vi "Configure List Save Or Recall.vi"(8 "error in":errorcluster, 9 "File Name":u8=1 min=1 max=10 step=1, 10 "Save Or Recall":u16(ring) items=["Save", "Recall"], 11 "VISA resource name":refnum<visa-resource-name>) -> (0 "error out":errorcluster, 3 "VISA resource name out":refnum<visa-resource-name>)   [LabVIEW 2018, in "IT-M3100.lvlib"]
doc: "This command is set to save or recall list file.\n<b>Save Or Recall</b>\n0:Save:This command saves the present list program into the specified memory.\n1:Recall:This command recalls the list program you saved in the specified memory location.\n<b>File Name</b>\n1-10"
uses:
  IT-M3100.lvlib
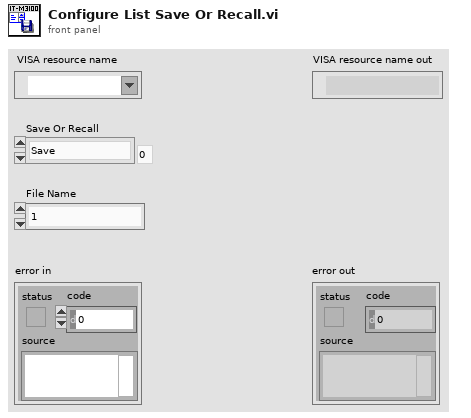
[diagram p1: front panel]
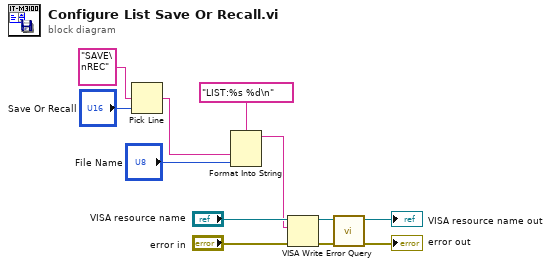
[diagram p0: block diagram]
diagram:
  n1 = Pick Line(multi-line string="SAVE\nREC", line index="Save Or Recall") -> (output string=w1:string)  [unwired: 1 in]
  n2 = Format Into String(format string="LIST:%s %d\n", w1, "File Name") -> (resulting string=w5:string)  [unwired: 2 in, 1 out]
  n3 = VISA Write(VISA resource name="VISA resource name", write buffer=w5, error in (no error)="error in") -> (VISA resource name out=w9:refnum<visa-resource-name>, error out=w10:errorcluster)  [unwired: 1 out]
  n4 = call "Error Query.vi"("error in"=w10, "VISA resource name"=w9) -> ("error out"=→"error out":errorcluster, "VISA resource name out"=→"VISA resource name out":refnum<visa-resource-name>)  [unwired: 6 in, 2 out]
